vi "_Close.vi"(8 "error in":errorcluster, 11 "Device In":u64) -> (0 "error out":errorcluster, 3 "Device Out":u64)   [LabVIEW 2020, in "Phidget Common.lvlib"]
doc: "Closes a Public"
uses:
  <instrlib>/Phidgets/Phidget Common/Phidget Common.lvlib
  phidget22.dll
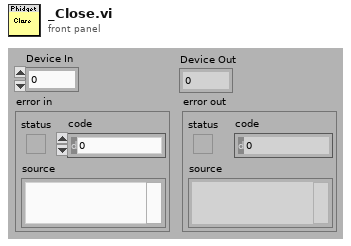
[diagram p1: front panel]
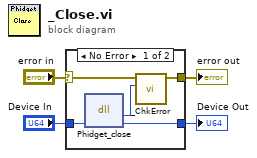
[diagram p0: block diagram]
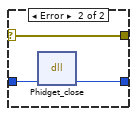
[diagram p2: hidden frame]
diagram:
  n1 = case shown="No Error" "error in" {
    selector: "error in" -> [w7 w12]
    tunnel: [w5 w12] -> w3
    tunnel: "Device In" -> [w9 w11]
    tunnel: [w8 w10] -> w1
    frame No Error {
      n2 = dll-call lib="phidget22.dll" fn="Phidget_close"("phid"=w9) -> ("return type"=w6:i32, "phid"=w8:u64)  [unwired: 3 in, 2 out]
      n3 = call <instrlib>:"_ChkError.vi"("Return Code"=w6, "error in (no error)"=w7) -> ("error out"=w5:errorcluster)  [unwired: 9 in]
    }
    frame Error {
      n4 = dll-call lib="phidget22.dll" fn="Phidget_close"("phid"=w11) -> ("phid"=w10:u64)  [unwired: 4 in, 2 out]
    }
  }
  "error out" <- w3
  "Device Out" <- w1
